vi "Replace_Array_Subset_2D.vi"(7 "E or S RAS":T2, 8 "SubArray RAS":i8[](array[numeric])=[-1, -2, -3], 9 "Element RAS":i8=-10, 10 "Indexs RAS":T1={"Rows"=-1, "Columns"=-1} {"Columns" min=-1; "Rows" min=-1}, 11 "RAS2D":i8[][](array[numeric])=[[0, 4, 7], [0, 5, 8], [3, 6, 9]]) -> (3 "New Array RAS2D":i8[][](array[numeric]))   [LabVIEW 2018]
uses:
  Controls/E_S.ctl
  Controls/Rows_Columns.ctl
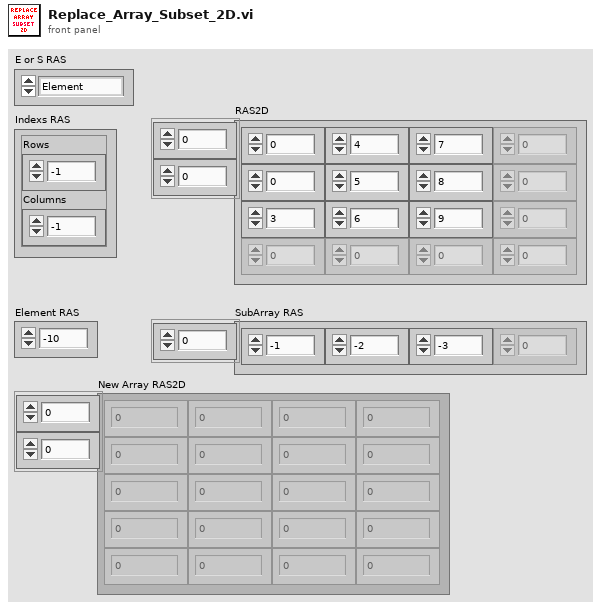
[diagram p1: front panel]
types:
  T1 = typedef "Rows_Columns.ctl" = cluster{"Rows":i32, "Columns":i32}
  T2 = typedef "E_S.ctl" = enum16{"Element", "SubArray"}
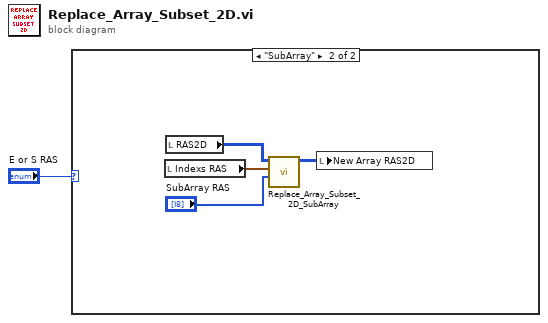
[diagram p0: block diagram]
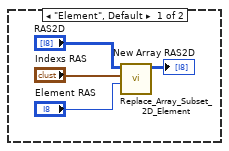
[diagram p2: hidden frame]
diagram:
  n1 = case shown="\"SubArray\"" "E or S RAS" {
    frame "Element", Default {
      n2 = call "Replace_Array_Subset_2D_Element.vi"("Element RAS"="Element RAS", "Indexs RAS"="Indexs RAS", "RAS2D"="RAS2D") -> ("New Array RAS2D"=→"New Array RAS2D":i8[][])  [unwired: 8 in]
    }
    frame "SubArray" {
      n3 = local read "Indexs RAS"() -> (w7:T1)
      n4 = local read "RAS2D"() -> (w8:i8[][])
      n5 = call "Replace_Array_Subset_2D_SubArray.vi"("SubArray RAS2D"="SubArray RAS", "Indexs RAS2D"=w7, "RAS2D"=w8) -> ("New Array RAS2D"=w9:i8[][])  [unwired: 8 in]
      n6 = local write "New Array RAS2D"(w9) -> ()
    }
  }
